vi "List Parts.vi"(4 "Region":T1, 7 "Request parameters":T6={"Max parts"=-1, "Part number marker"=1} {"Part number marker" min=1 max=10000; "Max parts" max=1000}, 8 "error in (no error)":errorcluster, 9 "Bucket":string, 10 "Object Path":string, 11 "Upload ID":string) -> (0 "error out":errorcluster, 3 "ListPartsResult":T2 {"Parts"."PartNumber" min=1 max=10000})   [LabVIEW 2015, in "LV Interface for Amazon S3.lvlib"]
doc: "This operation <B>lists the parts that have been uploaded</B> for a specific multipart upload. This operation <B>must include the upload ID</B>, which you obtain <B>by calling Get Multipart Upload ID.vi</B>."
uses:
  LV Interface for Amazon S3.lvlib
  Typedefs/AMZ_S3_API_List Parts Request Parameters.ctl
  Typedefs/AMZ_S3_API_ListPartsResult.ctl
  Typedefs/AMZ_S3_API_Owner.ctl
  Typedefs/AMZ_S3_Storage Class.ctl
  Typedefs/AMZ_S3_Multipart Upload Part Data.ctl
  Typedefs/AMZ_S3_LocationConstraint.ctl
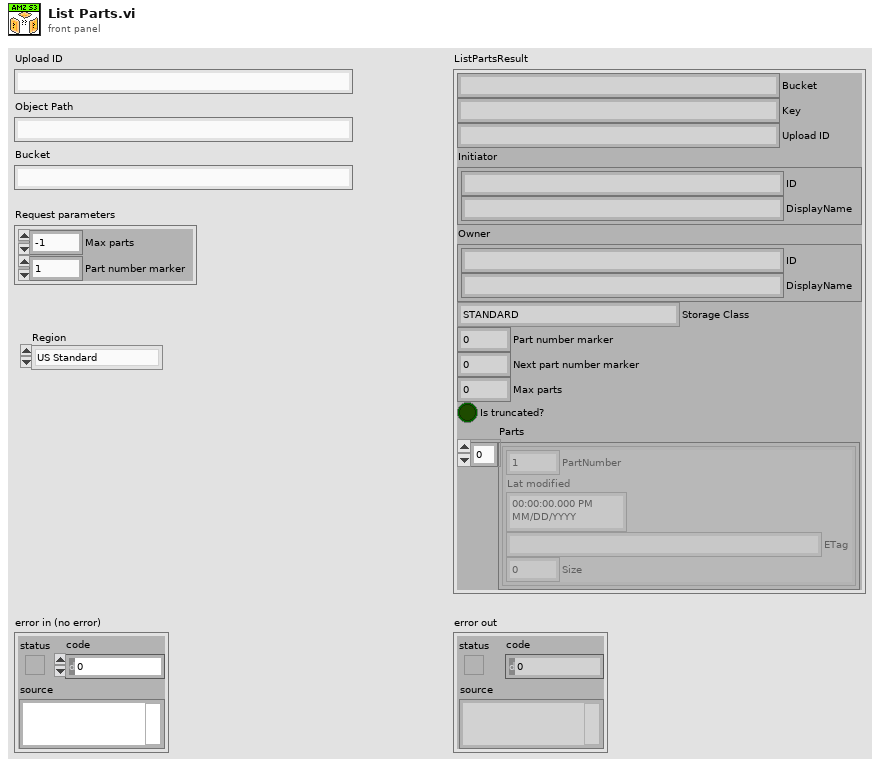
[diagram p1: front panel]
types:
  T1 = typedef "LV Interface for Amazon S3.lvlib/AMZ_S3_LocationConstraint.ctl" = enum16{"US Standard", "us-east-2", "us-west-1", "us-west-2", "ap-northeast-1", "ap-northeast-2", "ap-southeast-1", "ap-southeast-2", "ca-central-1", "eu-central-1", "eu-west-1", "eu-west-2", "sa-east-1"}
  T2 = typedef "LV Interface for Amazon S3.lvlib/AMZ_S3_API_ListPartsResult.ctl" = cluster{"Bucket":string, "Key":string, "Upload ID":string, "Initiator":T3, "Owner":T3, "Storage Class":T4, "Part number marker":u16, "Next part number marker":u16, "Max parts":u16, "Is truncated?":bool, "Parts":T5[]}
  T3 = typedef "LV Interface for Amazon S3.lvlib/AMZ_S3_API_Owner.ctl" = cluster{"ID":string, "DisplayName":string}
  T4 = typedef "LV Interface for Amazon S3.lvlib/AMZ_S3_Storage Class.ctl" = enum16{"STANDARD", "REDUCED_REDUNDANCY"}
  T5 = typedef "LV Interface for Amazon S3.lvlib/AMZ_S3_Multipart Upload Part Data.ctl" = cluster{"PartNumber":u16, "Lat modified":timestamp, "ETag":string, "Size":u64}
  T6 = typedef "LV Interface for Amazon S3.lvlib/AMZ_S3_API_List Parts Request Parameters.ctl" = cluster{"Max parts":i16, "Part number marker":u16}
  T7 = cluster{"format string":string, "Upload ID":string}
  T8 = cluster{"format string":string, "Upload ID":string}[]
  T9 = typedef "LV Interface for Amazon S3.lvlib/AMZ_S3_Call Results.ctl" = enum16{"Success", "UndefinedError", "AccessDenied", "AccountProblem", "AmbiguousGrantByEmailAddress", "BadDigest", "BucketAlreadyExists", "BucketAlreadyOwnedByYou", "BucketNotEmpty", "CredentialsNotSupported", "CrossLocationLoggingProhibited", "EntityTooSmall", "EntityTooLarge", "ExpiredToken", "IllegalVersioningConfigurationException", "IncompleteBody", "IncorrectNumberOfFilesInPostRequest", "InlineDataTooLarge", "InternalError", "InvalidAccessKeyId", "InvalidAddressingHeader", "InvalidArgument", "InvalidBucketName", "InvalidDigest", "InvalidLocationConstraint", "InvalidPart", "InvalidPartOrder", "InvalidPayer", "InvalidPolicyDocument", "InvalidRange", "InvalidSecurity", "InvalidSOAPRequest", "InvalidStorageClass", "InvalidTargetBucketForLogging", "InvalidToken", "InvalidURI", "KeyTooLong", "MalformedACLError", "MalformedPOSTRequest", "MalformedXML", "MaxMessageLengthExceeded", "MaxPostPreDataLengthExceededError", "MetadataTooLarge", "MethodNotAllowed", "MissingAttachment", "MissingContentLength", "MissingRequestBodyError", "MissingSecurityElement", "MissingSecurityHeader", "NoLoggingStatusForKey", "NoSuchBucket", "NoSuchKey", "NoSuchUpload", "NoSuchVersion", "NotImplemented", "NotSignedUp", "OperationAborted", "PermanentRedirect", "PreconditionFailed", "Redirect", "RequestIsNotMultiPartContent", "RequestTimeout", "RequestTimeTooSkewed", "RequestTorrentOfBucketError", "SignatureDoesNotMatch", "SlowDown", "TemporaryRedirect", "TokenRefreshRequired", "TooManyBuckets", "UnexpectedContent", "UnresolvableGrantByEmailAddress", "UserKeyMustBeSpecified", "LabVIEWError"}
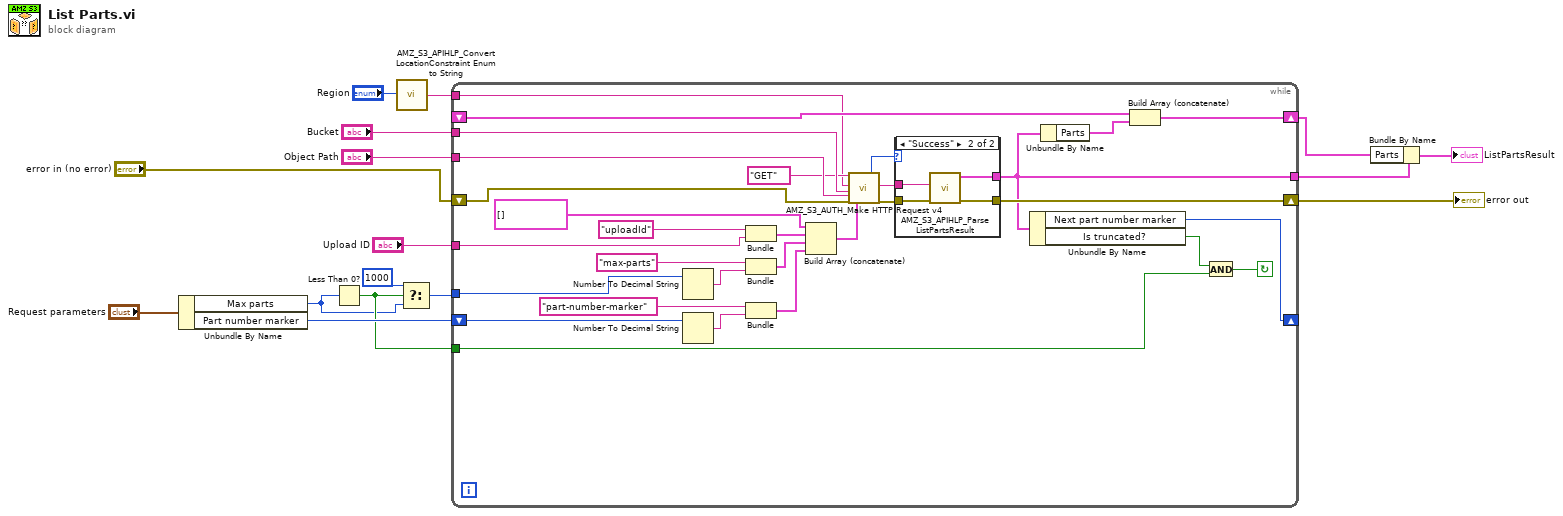
[diagram p0: block diagram]
diagram:
  n1 = Unbundle By Name("Request parameters") -> ("Max parts"=w9:i16, "Part number marker"=w14:u16)
  n2 = Less Than 0?(x=w9) -> (x < 0?=w10:bool)
  n3 = call "AMZ_S3_APIHLP_Convert LocationConstraint Enum to String.vi"("Location"="Region") -> ("Location String"=w1:string)  [unwired: 4 in]
  n4 = Select(t=i16 1000, s=w10, f=w9) -> (s? t:f=w8:i16)
  n5 = while {
    tunnel: "Object Path" -> [w34]
    tunnel: "Upload ID" -> [w28]
    tunnel: "Bucket" -> [w35]
    tunnel: [w43] -> w6
    shift-right: [w46] -> w11
    shift-left: "error in (no error)" -> [w19]
    shift-right: [w39] -> _
    shift-left: w14 -> [w22]
    tunnel: w10 -> [w21]
    tunnel: w8 -> [w26]
    shift-right: [w41] -> w4
    shift-left: _ -> [w40]
    tunnel: w1 -> [w17]
    stop <- w44 continue-if-true
    n6 = Number To Decimal String(number=w26) -> (decimal integer string=w30:string)  [unwired: 1 in]
    n7 = Number To Decimal String(number=w22) -> (decimal integer string=w24:string)  [unwired: 1 in]
    n8 = Bundle("format string"="uploadId", "Upload ID"=w28) -> (w29:T7)  [unwired: 1 in]
    n9 = Bundle("format string"="max-parts", w30) -> (w27:cluster{"format string":string, string})  [unwired: 1 in]
    n10 = Bundle("format string"="part-number-marker", w24) -> (w23:cluster{"format string":string, string})  [unwired: 1 in]
    n11 = Build Array (concatenate)(cluster{"item":string, "value":string}[] [] ("request parameters"), w29, w27, w23) -> (w20:T8)
    n12 = call "AMZ_S3_AUTH_Make HTTP Request v4.vi"("HTTP-Verb"="GET", "Region"=w17, "Bucket"=w35, "Object Key"=w34, "error in"=w19, "request parameters"=w20) -> ("Call Result"=w38:T9, "response body"=w37:string, "error out"=w36:errorcluster)  [unwired: 10 in, 1 out]
    n13 = case shown="\"Success\"" w38 {
      tunnel: w36 -> [w47 w51]
      tunnel: w37 -> [_ w50]
      tunnel: [_ w49] -> w43
      tunnel: [w47 w48] -> w46
      frame Default {
      }
      frame "Success" {
        n14 = call "AMZ_S3_APIHLP_Parse ListPartsResult.vi"("error in (no error)"=w51, "Response body"=w50) -> ("error out"=w48:errorcluster, "ListPartsResult"=w49:T2)  [unwired: 8 in]
      }
    }
    n15 = Unbundle By Name(w43) -> ("Next part number marker"=w39:u16, "Is truncated?"=w45:bool)
    n16 = Unbundle By Name(w43) -> ("Parts"=w42:T5[])
    n17 = Build Array (concatenate)(w40, w42) -> (w41:T5[])
    n18 = And(x=w45, y=w21) -> (x .and. y?=w44:bool)
  }
  "error out" <- w11
  n19 = Bundle By Name(cluster=w6, "Parts"=w4) -> (→"ListPartsResult":T2)
